vi "Init.vi"(8 "error in":errorcluster, 11 "Plugin_Controller in":refnum<class "Plugin_Controller.lvclass">) -> (0 "error out":errorcluster, 3 "Plugin_Controller out":refnum<class "Plugin_Controller.lvclass">)   [LabVIEW 2020, in "Plugin.lvlib" / "Plugin_Controller.lvclass"]
doc: "This VI executes while starting the test execution with the Plugin."
uses:
  Plugin_Controller.lvclass
  C:/SVN_LabSys/labsys_lvcode/LabSys_SourceCode/builds/Libraries/LabSys Framework.lvlibp/Configurable Data Node/Configurable Data Node/Configurable Data Node.lvclass
  C:/SVN_LabSys/labsys_lvcode/LabSys_SourceCode/builds/Libraries/LabSys Framework.lvlibp/Data Node/Data Node/Data Node.lvclass
  C:/SVN_LabSys/labsys_lvcode/LabSys_SourceCode/builds/Libraries/LabSys Framework.lvlibp/Devices/Device Driver.lvclass
  Typedefs/Connection type.ctl
  Drivers/Instrument Driver/VISA Interface/VISA Interface.lvclass
  C:/SVN_LabSys/labsys_lvcode/LabSys_SourceCode/Plugin Template/Source/Drivers/Instrument Driver/Instrument Driver.lvclass
  builds/Libraries/Value Object Library.lvlibp/Double/Double.lvclass
  C:/SVN_LabSys/labsys_lvcode/LabSys_SourceCode/builds/Libraries/LabSys Framework.lvlibp/Data Distributor/Value/Value.lvclass
  builds/Libraries/LabSys Framework.lvlibp/Data Distributor/Value/Value Status.ctl
  builds/Libraries/LabSys Framework.lvlibp/Data Distributor/Data Distributor/Value Update.ctl
  builds/Libraries/LabSys Framework.lvlibp/Data Distributor/Value/Value.lvclass
  Drivers/Instrument Driver/Typedefs/Output Settings.ctl
  Channels/Output Channels/Output Channels.lvclass
  C:/SVN_LabSys/labsys_lvcode/LabSys_SourceCode/Plugin Template/Source/Code/Channels/Plugin_Channels.lvclass
  builds/Libraries/LabSys Framework.lvlibp/Configurable Data Node/Configurable Data Node/Read Module Configuration.vi
  builds/Libraries/LabSys Framework.lvlibp/Data Node/Data Node/Read Error Manager.vi
  builds/Libraries/LabSys Framework.lvlibp/Configuration Storage/Module Configuration/Read Module Name.vi
  builds/Libraries/Value Object Library.lvlibp/Double/Write Value.vi
  builds/Libraries/LabSys Framework.lvlibp/Data Distributor/Value/Write Status.vi
  builds/Libraries/LabSys Framework.lvlibp/Data Distributor/Value/Write Time Stamp.vi
  builds/Libraries/LabSys Framework.lvlibp/Configuration Storage/Module Configuration/Module Configuration.lvclass
  Plugin_Driver/Plugin_Driver.lvclass
  builds/Libraries/LabSys Framework.lvlibp/Error Manager/Error Manager/Error Manager.lvclass
  Drivers/Instrument Driver/UDP/UDP.lvclass
  Drivers/Instrument Driver/UDP/Typedefs/Device Details.ctl
  UI_Class/Plugin_UI.lvclass
  Drivers/Instrument Driver/Instrument Driver.lvclass
  builds/Libraries/LabSys Framework.lvlibp/Data Node/Data Node/Data Node.lvclass
  builds/Libraries/LabSys Framework.lvlibp/Data Distributor/Data Distributor/Data Distributor.lvclass
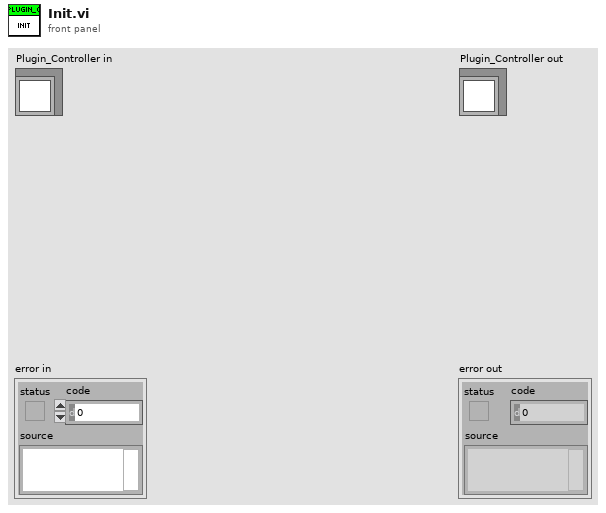
[diagram p1: front panel]
types:
  T1 = typedef "LabSys Framework.lvlibp/Data Distributor.lvlib/Data Distributor.lvclass/Value Update.ctl" = cluster{"Variable Name":string, "Value":refnum<class "Value.lvclass">}
  T2 = typedef "LabSys Framework.lvlibp/Data Distributor.lvlib/Value.lvclass/Value Status.ctl" = enum8{"FAIL", "OK", "UNDEFINED"}
  T3 = typedef "Plugin Instrument Driver.lvlib/Instrument Driver.lvclass/Output Settings.ctl" = cluster{"Voltage (V)":dbl}
  T4 = typedef "Plugin Instrument Driver.lvlib/UDP.lvclass/Device Details.ctl" = cluster{"Device Port Number":u16, "Device IP":string, "Timeout":i32, "Port Number":u16, "Connection ID":refnum<k16>}
  T5 = typedef "Plugin.lvlib/Plugin_Controller.lvclass/Connection type.ctl" = enum16{"Serial", "UDP"}
  T6 = typedef "Plugin.lvlib/Plugin_UI.lvclass/Serial Configuration.ctl" = cluster{"VISA":refnum<visa-resource-name>, "Interface Type":T7, "Serial Interface":T8, "Slave Address":u8}
  T7 = typedef "Shared GUI Library.lvlibp/Interface Type.ctl" = u16
  T8 = typedef "Shared GUI Library.lvlibp/Serial Interafce.ctl" = cluster{"Baud Rate":u32, "Data Bits ":u16, "Parity":enum16{"None", "Odd", "Even"}, "Stop Bits":u16}
  T9 = typedef "Plugin.lvlib/Plugin_UI.lvclass/UDP Configuration.ctl" = cluster{"Device Port Number":u16, "Device IP":string, "Timeout":i32, "Port Number":u16}
  T10 = typedef "Shared GUI Library.lvlibp/Get Meta Data.ctl" = cluster{"Serial Number":string, "Firmware":string, "Model Number":string, "Manufacturer":string, "Calibration Date":string}
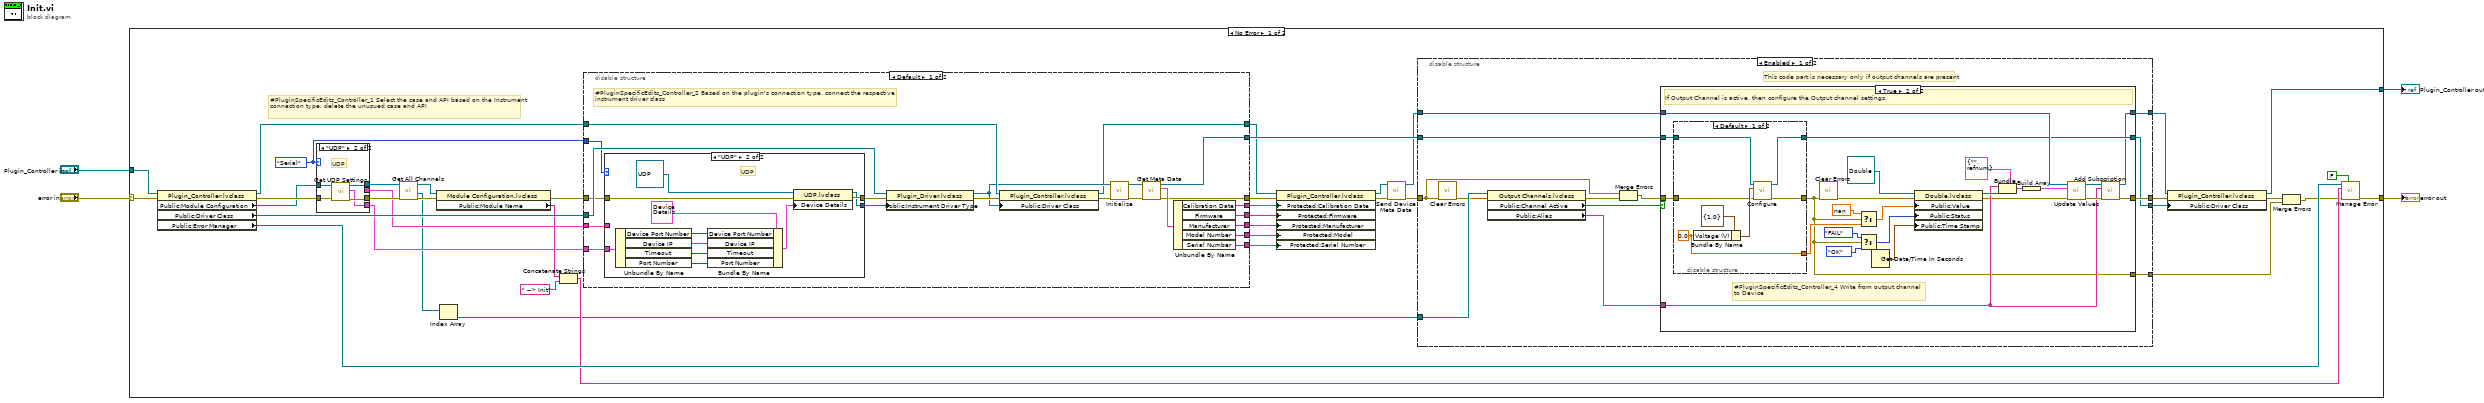
[diagram p0: block diagram]
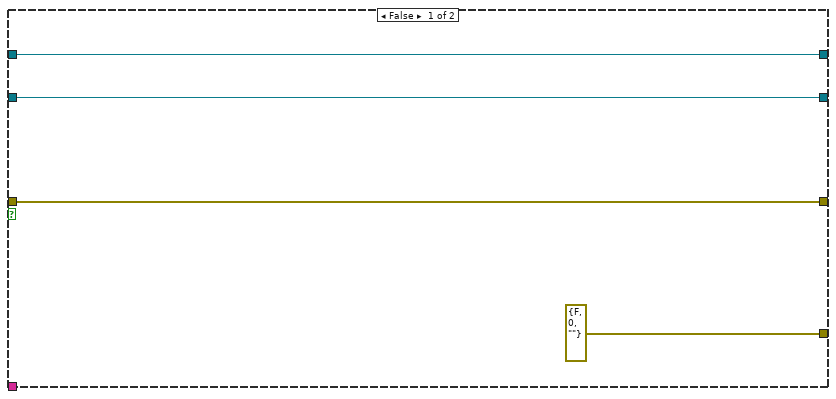
[diagram p2: hidden frame]
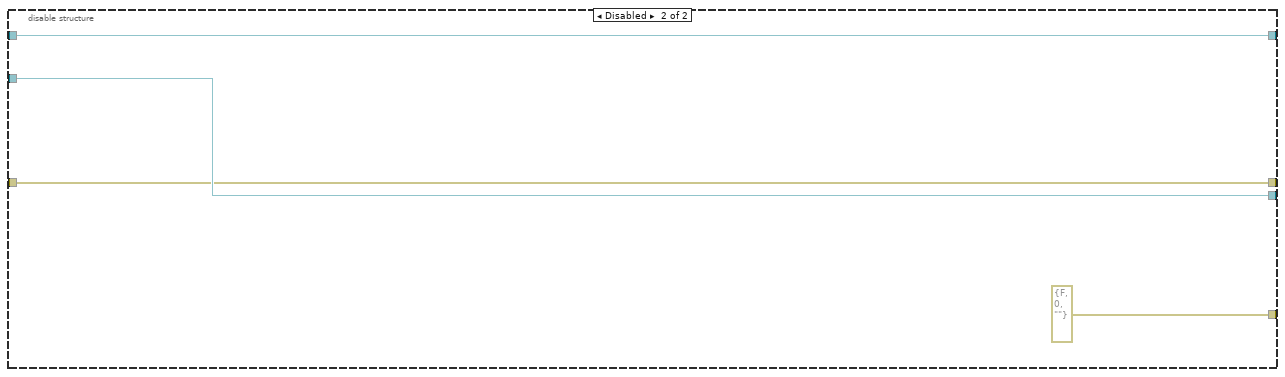
[diagram p4: hidden frame]
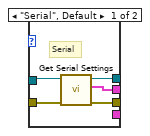
[diagram p5: hidden frame]
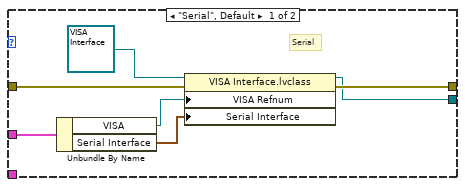
[diagram p6: hidden frame]
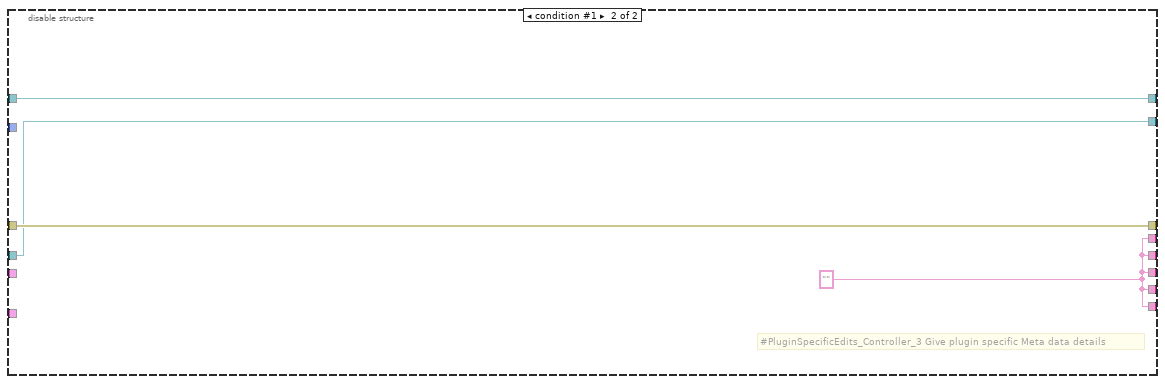
[diagram p7: hidden frame]
diagram:
  n1 = case shown="No Error" "error in" {
    selector: "error in" -> [w43 w155]
    tunnel: [w45 w155] -> w3
    tunnel: [w7 w154] -> w1
    tunnel: "Plugin_Controller in" -> [w44 w154]
    frame No Error {
      w27 = Connection_type."Serial" ("Connection Type")
      # "#PluginSpecificEdits_Controller_1 Select the case and API based on the Instrument connection type, delete the unusued case and API"
      n2 = property on="Property Node" class="Plugin_Controller.lvclass"(reference=w44, error in=w43) -> (reference out=w6:refnum<class "Plugin_Controller.lvclass">, error out=w33:errorcluster, "Public:Module Configuration"=w32:refnum<class "Module Configuration.lvclass">, "Public:Driver Class"=w41:refnum<class "Plugin_Driver.lvclass">, "Public:Error Manager"=w42:refnum<data-value>)
      n3 = case shown="\"UDP\"" w27 {
        tunnel: w33 -> [w104 w108]
        tunnel: w32 -> [w100 w109]
        tunnel: [w103 w105] -> w31
        tunnel: [w102 w107] -> w30
        tunnel: [w101 _] -> w29
        tunnel: [_ w106] -> w28
        frame "Serial", Default {
          # "Serial"
          n4 = call "Get Serial Settings.vi"("error IO"=w104, "Module Configuration in"=w100) -> ("error IO Out"=w102:errorcluster, "Serial Configuration"=w101:T6, "Module Configuration out"=w103:refnum<class "Module Configuration.lvclass">)  [unwired: 7 in]
        }
        frame "UDP" {
          # "UDP"
          n5 = call "Get UDP Settings.vi"("error in (no error)"=w108, "Module Configuration"=w109) -> ("error out"=w107:errorcluster, "UDP configuration"=w106:T9, "Module Configuration out"=w105:refnum<class "Module Configuration.lvclass">)  [unwired: 7 in]
        }
      }
      n6 = call "Get All Channels.vi"("error in (no error)"=w30, "Module Configuration"=w31) -> ("error out"=w34:errorcluster, "Output Channels[]"=w18:refnum<class "Output Channels.lvclass">[], "Module Configuration out"=w35:refnum<class "Module Configuration.lvclass">)  [unwired: 5 in, 2 out]
      n7 = property on="Property Node" class="Module Configuration.lvclass"(reference=w35, error in=w34) -> (error out=w40:errorcluster, "Public:Module Name"=w38:string)  [unwired: 1 out]
      n8 = Index Array(array=w18) -> (element=w17:refnum<class "Output Channels.lvclass">)  [unwired: 1 in]
      n9 = Concatenate Strings(w38, " --> Init" ("string")) -> (w37:string)
      n10 = disable-structure "Conditional Disable Structure" shown="Default" {
        disable-tunnel: w40 -> [w128 w153]
        disable-tunnel: [w122 w153] -> w26
        disable-tunnel: w41 -> [w131 w152]
        disable-tunnel: w29 -> [w126 _]
        disable-tunnel: w28 -> [w124 _]
        disable-tunnel: w27 -> [w125 _]
        disable-tunnel: [w121 w152] -> w15
        disable-tunnel: [w120 w151] -> w24
        disable-tunnel: [w119 w151] -> w23
        disable-tunnel: [w118 w151] -> w22
        disable-tunnel: [w117 w151] -> w21
        disable-tunnel: [w116 w151] -> w20
        disable-tunnel: w6 -> [w113 w150]
        disable-tunnel: [w110 w150] -> w5
        frame condition #0 (active) {
          # "#PluginSpecificEdits_Controller_2 Based on the plugin's connection type, connect the respective \ninstrument driver class"
          n11 = case shown="\"UDP\"" w125 {
            tunnel: w128 -> [w138 w142]
            tunnel: [w137 w141] -> w127
            tunnel: [w136 w140] -> w112
            tunnel: w126 -> [w135 _]
            tunnel: w124 -> [_ w139]
            frame "Serial", Default {
              # "Serial"
              n12 = Unbundle By Name(w135) -> ("VISA"=w133:refnum<visa-resource-name>, "Serial Interface"=w132:T8)
              n13 = property on="Property Node" class="VISA Interface.lvclass"(reference=refnum<class "VISA Interface.lvclass"> refnum ("Plugin Instrument Driver.lvlib:VISA Interface.lvclass"), error in=w138, "VISA Refnum"=w133, "Serial Interface"=w132) -> (reference out=w136:refnum<class "VISA Interface.lvclass">, error out=w137:errorcluster)
            }
            frame "UDP" {
              # "UDP"
              n14 = Unbundle By Name(w139) -> ("Device Port Number"=w147:u16, "Device IP"=w146:string, "Timeout"=w145:i32, "Port Number"=w144:u16)
              n15 = Bundle By Name(cluster=T4 {"Device Port Number"=2001, "Device IP"="192.168.1.1.100", "Timeout"=5000, "Port Number"=1234, "Connection ID"=refnum} ("Device Details"), "Device Port Number"=w147, "Device IP"=w146, "Timeout"=w145, "Port Number"=w144) -> (w143:T4)
              n16 = property on="Property Node" class="UDP.lvclass"(reference=refnum<class "UDP.lvclass"> refnum ("Plugin Instrument Driver.lvlib:UDP.lvclass"), error in=w142, "Device Details"=w143) -> (reference out=w140:refnum<class "UDP.lvclass">, error out=w141:errorcluster)
            }
          }
          n17 = property on="Property Node" class="Plugin_Driver.lvclass"(reference=w131, error in=w127, "Public:Instrument Driver Type"=w112) -> (reference out=w111:refnum<class "Plugin_Driver.lvclass">, error out=w115:errorcluster)
          n18 = property on="Property Node" class="Plugin_Controller.lvclass"(reference=w113, error in=w115, "Public:Driver Class"=w111) -> (reference out=w110:refnum<class "Plugin_Controller.lvclass">, error out=w114:errorcluster)
          n19 = call "Initialize.vi"("error in"=w114, "Plugin_Driver in"=w111) -> ("error out"=w129:errorcluster, "Plugin_Driver out"=w130:refnum<class "Plugin_Driver.lvclass">)  [unwired: 8 in]
          n20 = call "Get Meta Data.vi"("error in"=w129, "Plugin_Driver in"=w130) -> ("error out"=w122:errorcluster, "Get Meta Data"=w123:T10, "Plugin_Driver out"=w121:refnum<class "Plugin_Driver.lvclass">)  [unwired: 7 in]
          n21 = Unbundle By Name(w123) -> ("Calibration Date"=w120:string, "Firmware"=w119:string, "Manufacturer"=w118:string, "Model Number"=w117:string, "Serial Number"=w116:string)
        }
        frame condition #1 {
          w151 = "" ("Calibration Date")
          # "#PluginSpecificEdits_Controller_3 Give plugin specific Meta data details"
        }
      }
      n22 = property on="Property Node" class="Plugin_Controller.lvclass"(reference=w5, error in=w26, "Protected:Calibration Date"=w24, "Protected:Firmware"=w23, "Protected:Manufacturer"=w22, "Protected:Model"=w21, "Protected:Serial Number"=w20) -> (reference out=w25:refnum<class "Plugin_Controller.lvclass">, error out=w19:errorcluster)
      n23 = call "Send Device Meta Data.vi"("error in"=w19, "Plugin_Controller in"=w25) -> ("error out"=w16:errorcluster, "Plugin_Controller out"=w14:refnum<class "Plugin_Controller.lvclass">)  [unwired: 8 in]
      n24 = disable-structure "Diagram Disable Structure" shown="Enabled" {
        disable-tunnel: w17 -> [w58 _]
        disable-tunnel: w16 -> [w48 w97]
        disable-tunnel: w15 -> [w56 w98]
        disable-tunnel: w14 -> [w55 w99]
        disable-tunnel: [w53 w97] -> w13
        disable-tunnel: [w52 w99] -> w12
        disable-tunnel: [w51 w98] -> w11
        disable-tunnel: [w50 errorcluster {"status"=FALSE, "code"=0, "source"=""} ("error out")] -> w9
        frame Enabled {
          # "This code part is necessary only if output channels are present"
          n25 = call <vilib>:"Clear Errors.vi"("error in (no error)"=w48) -> ("error out"=w49:errorcluster)  [unwired: 5 in, 1 out]
          n26 = property on="Property Node" class="Output Channels.lvclass"(reference=w58, error in=w49) -> (error out=w47:errorcluster, "Public:Channel Active"=w57:bool, "Public:Alias"=w54:string)  [unwired: 1 out]
          n27 = Merge Errors(w48, w47) -> (w46:errorcluster)
          n28 = case shown="True" w57 {
            tunnel: w46 -> [w61 w86]
            tunnel: w56 -> [w62 w85]
            tunnel: w55 -> [w60 w72]
            tunnel: w54 -> [_ w69]
            tunnel: [errorcluster {"status"=FALSE, "code"=0, "source"=""} ("error out") w67] -> w50
            tunnel: [w61 w66] -> w53
            tunnel: [w62 w65] -> w51
            tunnel: [w60 w64] -> w52
            frame False {
            }
            frame True {
              # "#PluginSpecificEdits_Controller_4 Write from output channel\nto Device"
              # "If Output Channel is active, then configure the Output channel settings."
              n29 = disable-structure "Conditional Disable Structure" shown="Default" {
                disable-tunnel: w86 -> [w91 w94]
                disable-tunnel: w85 -> [w90 w95]
                disable-tunnel: [w89 w94] -> w67
                disable-tunnel: [w88 w95] -> w65
                disable-tunnel: [w87 _] -> w71
                frame condition #0 (active) {
                  w87 = 0.0 ("Voltage (V)")
                  n30 = Bundle By Name(cluster=T3 {"Voltage (V)"=1.0} ("Output Settings"), "Voltage (V)"=w87) -> (w92:T3)
                  n31 = call "Configure.vi"("error in"=w91, "Output Settings"=w92, "Plugin_Driver in"=w90) -> ("error out"=w89:errorcluster, "Plugin_Driver out"=w88:refnum<class "Plugin_Driver.lvclass">)  [unwired: 7 in]
                }
                frame condition #1 {
                }
              }
              n32 = call <vilib>:"Clear Errors.vi"("error in (no error)"=w67) -> ("error out"=w75:errorcluster)  [unwired: 5 in, 1 out]
              n33 = Select(t=nan, s=w67, f=w71) -> (s? t:f=w83:dbl)
              n34 = Select(t=Value_Status."FAIL" ("Status"), s=w67, f=Value_Status."OK" ("Status")) -> (s? t:f=w82:T2)
              n35 = Get Date/Time In Seconds() -> (seconds since 1Jan1904=w84:timestamp)
              n36 = property on="Property Node" class="Double.lvclass"(reference=refnum<class "Double.lvclass"> refnum ("Value Object Library.lvlibp:Double.lvclass"), error in=w75, "Public:Value"=w83, "Public:Status"=w82, "Public:Time Stamp"=w84) -> (reference out=w81:refnum<class "Double.lvclass">, error out=w63:errorcluster)
              n37 = Bundle(cluster=T1 {"Variable Name"="", "Value"=refnum} ("Value Update"), "Variable Name"=w69, "Value"=w81) -> (w74:T1)
              n38 = Build Array(w74) -> (w73:T1[])
              n39 = call "Update Values.vi"("error in (no error)"=w63, "Value Updates"=w73, "Data Node in"=w72) -> ("error out"=w70:errorcluster, "Data Node out"=w68:refnum<class "Plugin_Controller.lvclass">)  [unwired: 7 in]
              n40 = call-dynamic "Add Subscription.vi"("error in (no error)"=w70, "Variable Name"=w69, "Data Node in"=w68) -> ("error out"=w66:errorcluster, "Data Node out"=w64:refnum<class "Plugin_Controller.lvclass">)  [unwired: 7 in]
            }
          }
        }
        frame Disabled {
        }
      }
      n41 = property on="Property Node" class="Plugin_Controller.lvclass"(reference=w12, error in=w13, "Public:Driver Class"=w11) -> (reference out=w7:refnum<class "Plugin_Controller.lvclass">, error out=w10:errorcluster)
      n42 = Merge Errors(w10, w9) -> (w8:errorcluster)
      n43 = call "Manage Error.vi"("Clear Errors (F)"=FALSE, "error in (no error)"=w8, "Error Location"=w37, "Error Manager in"=w42) -> ("error out"=w45:errorcluster)  [unwired: 6 in, 1 out]
    }
    frame Error {
    }
  }
  "error out" <- w3
  "Plugin_Controller out" <- w1
